vi "GL_DRC_GPIBadd.vi"() -> ()   [LabVIEW 2024]
panel:
  in  "GPIB Address":string
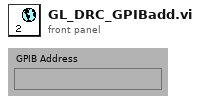
[diagram p1: front panel]
diagram:
